vi "SearchFoodInArray.vi"(2 "ID":i32, 3 "信息数组":cluster{"ID":dbl, "食品名称":string, "价格":dbl}[](array[cluster])) -> (0 "Found Index":i32, 1 "Exist?":bool)   [LabVIEW 2013, in "FoodBase.lvclass"]
doc: "在员工信息数组中查找具有指定员工编号的员工信息。\n\n如果找到，Finded Index为该员工在数组中的index。\n否则，Finded Index为-1"
uses:
  FoodBase.lvclass
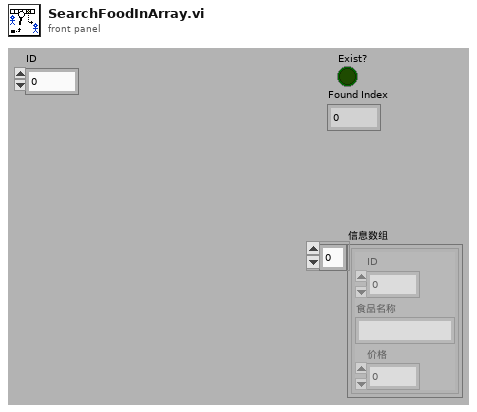
[diagram p1: front panel]
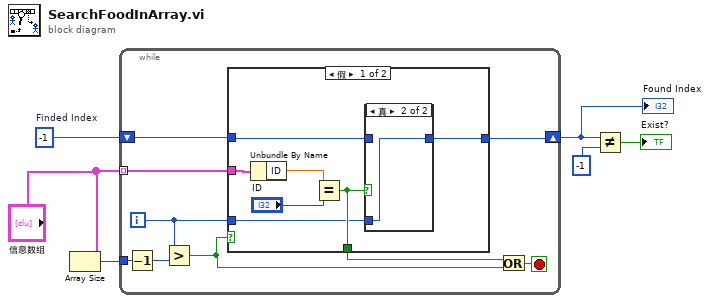
[diagram p0: block diagram]
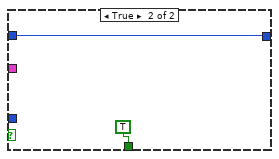
[diagram p3: hidden frame]
diagram:
  w5 = -1  # Finded Index
  n1 = Array Size(array="信息数组") -> (size(s)=w6:i32)
  n2 = while {
    tunnel: "信息数组" -> [w14] mode=indexing
    tunnel: w6 -> [w15]
    shift-right: [w8] -> w3
    shift-left: w5 -> [w9]
    i -> [w10]
    stop <- w12 stop-if-true
    n3 = Decrement(x=w15) -> (x-1=w13:i32)
    n4 = Greater?(x=w10, y=w13) -> (0:w7:bool)
    n5 = case shown="假" w7 {
      tunnel: w14 -> [w22 _]
      tunnel: [w21 TRUE] -> w11
      tunnel: w10 -> [w20 _]
      tunnel: w9 -> [w19 w26]
      tunnel: [w18 w26] -> w8
      frame False {
        n6 = Unbundle By Name(w22) -> ("ID"=w16:dbl)
        n7 = Equal?(x=w16, y="ID") -> (x = y?=w21:bool)
        n8 = case shown="真" w21 {
          tunnel: w20 -> [_ w24]
          tunnel: w19 -> [w23 _]
          tunnel: [w23 w24] -> w18
          frame False {
          }
          frame True {
          }
        }
      }
      frame True {
      }
    }
    n9 = Or(x=w11, y=w7) -> (x .or. y?=w12:bool)
  }
  "Found Index" <- w3
  n10 = Not Equal?(x=w3, y=-1 ("Finded Index")) -> (x != y?=→"Exist?":bool)
